vi "mj_getFormatExtDesc.vi"(11 "Data storage format":u16(ring) items=["TDM Streaming (high performance)", "TDM with XML Header (medium performance)"]) -> (2 "Format description":string, 3 "Format extension":string)   [LabVIEW 2020]
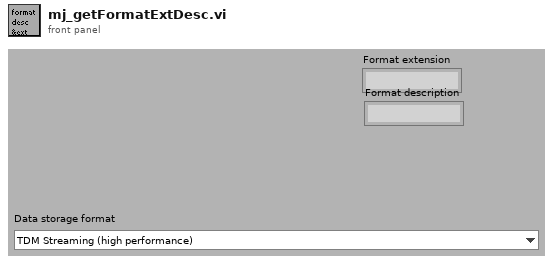
[diagram p1: front panel]
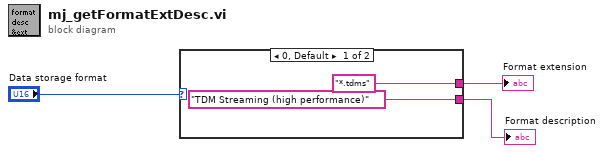
[diagram p0: block diagram]
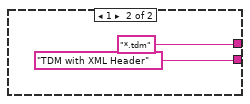
[diagram p2: hidden frame]
diagram:
  n1 = case shown="0, Default" "Data storage format" {
    tunnel: ["*.tdms" ("Browse Options:Match Pattern") "*.tdm" ("Browse Options:Match Pattern")] -> w2
    tunnel: ["TDM Streaming (high performance)" ("Browse Options:Pattern Label") "TDM with XML Header" ("Browse Options:Pattern Label")] -> w1
    frame 0, Default {
    }
    frame 1 {
    }
  }
  "Format extension" <- w2
  "Format description" <- w1
